vi "Telnet Listen.vi"(8 "error in (no error)":errorcluster, 9 "timeout ms (wait forever : -1)":i32=-1, 10 "port":u16) -> (0 "error out":errorcluster, 1 "remote port":u16, 2 "remote address":string, 3 "telnet connection":T1)   [LabVIEW 2011]
uses:
  Telnet Session.ctl
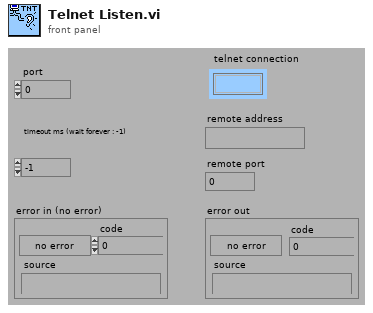
[diagram p1: front panel]
types:
  T1 = typedef "Telnet Session.ctl" = refnum<k1>
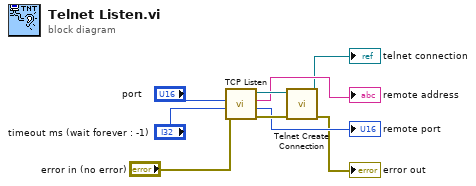
[diagram p0: block diagram]
diagram:
  n1 = call <vilib>:"TCP Listen.vi"("error in (no error)"="error in (no error)", "timeout ms (wait forever: -1)"="timeout ms (wait forever : -1)", "port"="port") -> ("error out"=w5:errorcluster, "remote port"=→"remote port":u16, "remote address"=→"remote address":string, "connection ID"=w6:refnum<k5>)  [unwired: 4 in, 1 out]
  n2 = call "Telnet Create Connection.vi"("error in (no error)"=w5, "TCP connection"=w6) -> ("error out"=→"error out":errorcluster, "telnet connection"=→"telnet connection":T1)  [unwired: 8 in]
